vi "Factory settings laden Messgeraet.vi"(0 "Ordner des Haupt-VIs":path, 4 "Dateiname":string="abc", 5 "Rolling Average Settings":T1={"Average"=1, "Average via AK:"=FALSE, "Average IAG Software:"=FALSE} {"Average" min=1 max=600}, 7 "error in (no error)":errorcluster caption="Fehler (Eingang, kein Fehler)", 8 "Startadresse":i32, 10 "Anzahl":i32, 12 "1Hz/5Hz Gerät":T2=1 items=["1Hz"=1, "5Hz"=5, "10Hz"=10], 14 "1Hz/5Hz Leitsystem":T2=1 items=["1Hz"=1, "5Hz"=5, "10Hz"=10], 18 "Smoothing?":bool) -> (20 "Startadresse":i32, 21 "Anzahl":i32, 22 "1Hz/5Hz Leitsystem":T2=1 items=["1Hz"=1, "5Hz"=5, "10Hz"=10], 23 "1Hz/5Hz Gerät":T2=1 items=["1Hz"=1, "5Hz"=5, "10Hz"=10], 25 "Rolling Average Settings":T1={"Average"=1, "Average via AK:"=FALSE, "Average IAG Software:"=FALSE} {"Average" min=1 max=600}, 26 "Smoothing?":bool, 27 "error out":errorcluster caption="Fehler (Ausgang)")   [LabVIEW 2020, in "allgemeine Sub-VIs.lvlib"]
uses:
  allgemeine Sub-VIs.lvlib
  Seiten/FT-IR/1Hz-5Hz Geraet.ctl
  <vilib>/Utility/config.llb/Read Key (I32).vi
  <vilib>/Utility/config.llb/Read Key (Boolean).vi
  <vilib>/Utility/config.llb/NI_LVConfig.lvlib
  <vilib>/Utility/config.llb/Read Key (U32).vi
  Seiten/FT-IR/FT-IR.lvlib
  Seiten/FT-IR/Rolling Average Settings.ctl
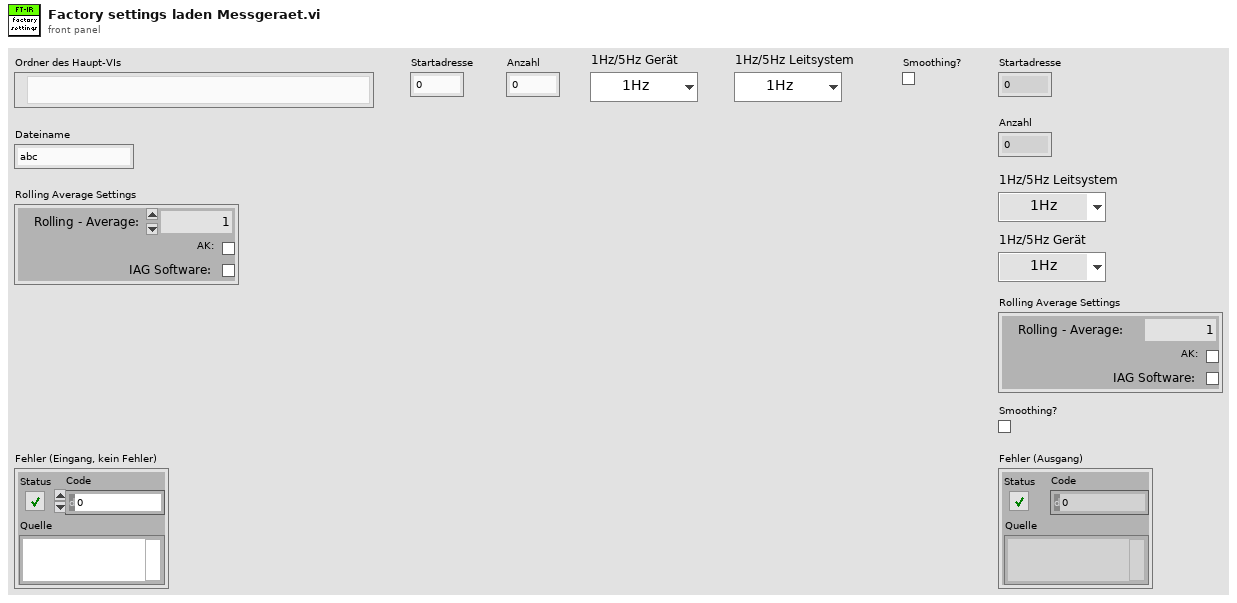
[diagram p1: front panel]
types:
  T1 = typedef "FT-IR.lvlib/Rolling Average Settings.ctl" = cluster{"Average":u32, "Average via AK:":bool, "Average IAG Software:":bool}
  T2 = typedef "FT-IR.lvlib/1Hz-5Hz Geraet.ctl" = u16
  T3 = typedef "NI_LVConfig.lvlib/Config Data RefNum.ctl" = refnum<k1>
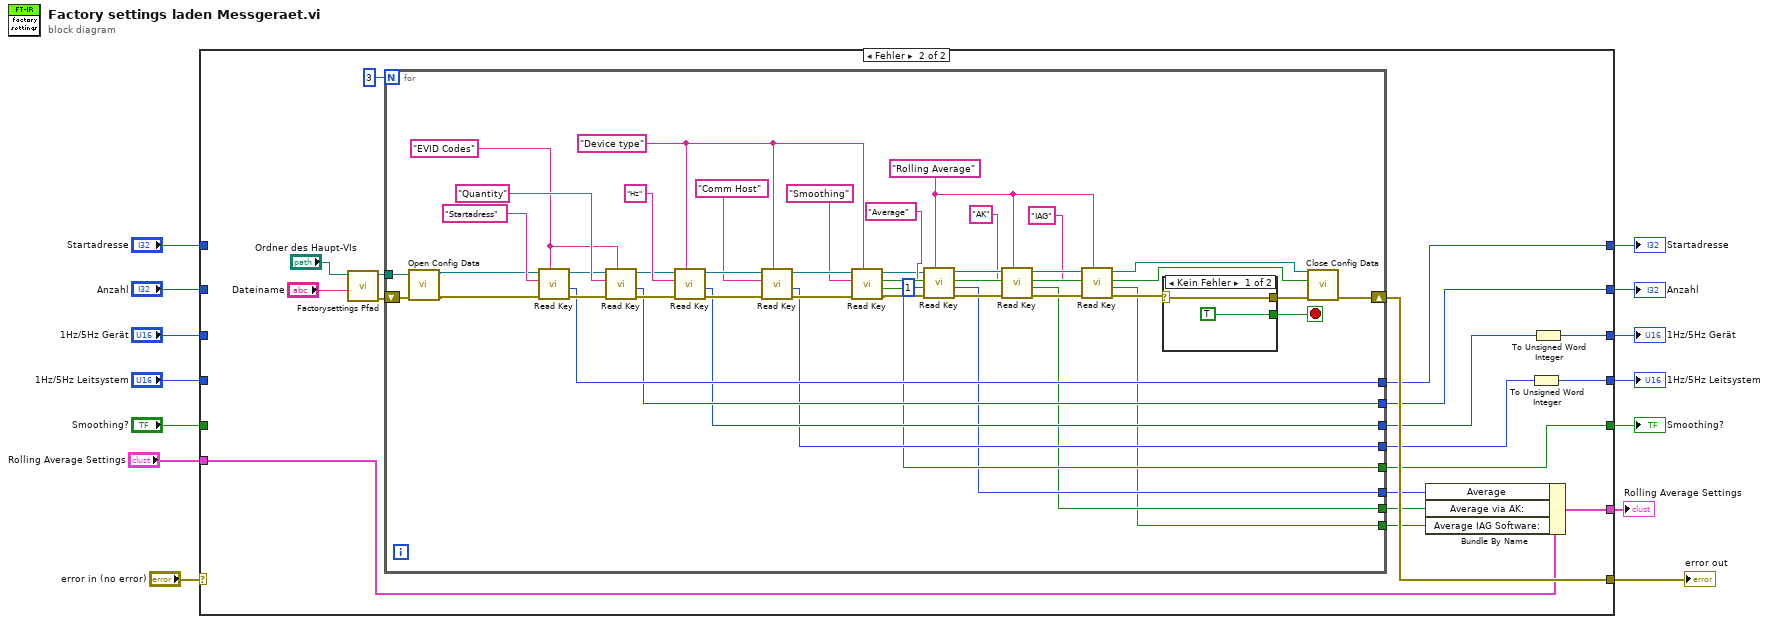
[diagram p0: block diagram]
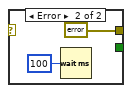
[diagram p3: hidden frame]
diagram:
  n1 = case shown="Fehler" "error in (no error)" {
    selector: "error in (no error)" -> [w21 _]
    tunnel: [w21 w39] -> w13
    tunnel: "Startadresse" -> [w20 _]
    tunnel: "Anzahl" -> [w19 _]
    tunnel: "1Hz/5Hz Gerät" -> [w18 _]
    tunnel: "1Hz/5Hz Leitsystem" -> [w17 _]
    tunnel: "Smoothing?" -> [w16 _]
    tunnel: [w20 w33] -> w7
    tunnel: [w19 w32] -> w5
    tunnel: [w18 w28] -> w4
    tunnel: [w17 w27] -> w3
    tunnel: [w16 w29] -> w6
    tunnel: "Rolling Average Settings" -> [w15 w26]
    tunnel: [w15 w22] -> w1
    frame No Error {
    }
    frame Error {
      n2 = call "Factorysettings Pfad.vi"("Dateiname"="Dateiname", "Ordner des Haupt-VIs"="Ordner des Haupt-VIs") -> ("error out"=w37:errorcluster, "Pfad Factorysettings"=w38:path)  [unwired: 8 in]
      n3 = for {
        N: 3 -> [_]
        tunnel: w38 -> [w82]
        shift-right: [w83] -> w39
        shift-left: w37 -> [w81]
        tunnel: [w60] -> w33
        tunnel: [w59] -> w32
        tunnel: [w58] -> w31
        tunnel: [w57] -> w30
        tunnel: [w56] -> w29
        tunnel: [w43] -> w25
        tunnel: [w41] -> w24
        tunnel: [w40] -> w23
        stop <- w79 stop-if-true
        w51 = "Rolling Average" ("section")
        w78 = "Device type" ("section")
        w66 = "EVID Codes" ("section")
        n4 = call <vilib>:"Open Config Data.vi"("error in (no error)"=w81, "configuration file path"=w82) -> ("error out"=w62:errorcluster, "refnum"=w63:T3)  [unwired: 7 in, 1 out]
        n5 = call-poly <vilib>:"Read Key.vi"("section"=w66, "error in (no error)"=w62, "key"="Startadress", "refnum"=w63) -> ("error out"=w64:errorcluster, "value"=w60:i32, "refnum out"=w65:T3)  [unwired: 4 in, 1 out]
        n6 = call-poly <vilib>:"Read Key.vi"("section"=w66, "error in (no error)"=w64, "key"="Quantity", "refnum"=w65) -> ("error out"=w70:errorcluster, "value"=w59:i32, "refnum out"=w69:T3)  [unwired: 4 in, 1 out]
        n7 = call-poly <vilib>:"Read Key.vi"("section"=w78, "error in (no error)"=w70, "key"="Hz", "refnum"=w69) -> ("error out"=w74:errorcluster, "value"=w58:i32, "refnum out"=w73:T3)  [unwired: 4 in, 1 out]
        n8 = call-poly <vilib>:"Read Key.vi"("section"=w78, "error in (no error)"=w74, "key"="Comm Host", "refnum"=w73) -> ("error out"=w77:errorcluster, "value"=w57:i32, "refnum out"=w76:T3)  [unwired: 4 in, 1 out]
        n9 = call-poly <vilib>:"Read Key.vi"("section"=w78, "error in (no error)"=w77, "key"="Smoothing", "refnum"=w76) -> ("error out"=w44:errorcluster, "value"=w56:bool, "found?"=w61:bool, "refnum out"=w45:T3)  [unwired: 4 in]
        n10 = call-poly <vilib>:"Read Key.vi"("section"=w51, "error in (no error)"=w44, "default value"=u32 1, "key"="Average" ("section"), "refnum"=w45) -> ("error out"=w55:errorcluster, "value"=w43:u32, "refnum out"=w54:T3)  [unwired: 3 in, 1 out]
        n11 = call-poly <vilib>:"Read Key.vi"("section"=w51, "error in (no error)"=w55, "key"="AK" ("section"), "refnum"=w54) -> ("error out"=w53:errorcluster, "value"=w41:bool, "refnum out"=w52:T3)  [unwired: 4 in, 1 out]
        n12 = call-poly <vilib>:"Read Key.vi"("section"=w51, "error in (no error)"=w53, "key"="IAG" ("section"), "refnum"=w52) -> ("error out"=w47:errorcluster, "value"=w40:bool, "refnum out"=w46:T3)  [unwired: 4 in, 1 out]
        n13 = case shown="Kein Fehler" w47 {
          selector: w47 -> [w85 _]
          tunnel: [w85 errorcluster {"status"=FALSE, "code"=0, "source"=""} ("error IO")] -> w80
          tunnel: [TRUE _] -> w79
          frame No Error {
          }
          frame Error {
            n14 = Wait (ms)(milliseconds to wait=u32 100 ("Zu wartende ms")) -> ()  [unwired: 1 out]
          }
        }
        n15 = call <vilib>:"Close Config Data.vi"("error in (no error)"=w80, "write file if changed (T)"=w61, "refnum"=w46) -> ("error out"=w83:errorcluster)  [unwired: 7 in, 1 out]
      }
      n16 = Bundle By Name(cluster=w26, "Average"=w25, "Average via AK:"=w24, "Average IAG Software:"=w23) -> (w22:T1)
      n17 = To Unsigned Word Integer(number=w30) -> (unsigned 16bit integer=w27:u16)
      n18 = To Unsigned Word Integer(number=w31) -> (unsigned 16bit integer=w28:u16)
    }
  }
  "error out" <- w13
  "Startadresse" <- w7
  "Anzahl" <- w5
  "1Hz/5Hz Gerät" <- w4
  "1Hz/5Hz Leitsystem" <- w3
  "Smoothing?" <- w6
  "Rolling Average Settings" <- w1
